vi "Read Dev Bounds.vi"(8 "error in (no error)":errorcluster, 11 "VISA resource name":refnum<visa-resource-name>) -> (0 "error out":errorcluster, 2 "dev bounds":T1, 3 "VISA resource name out":refnum<visa-resource-name>)   [LabVIEW 2019, in "Andeen-Hagerling 2700A.lvlib"]
doc: "Return the value of the deviation mode bounds parameters.\n\nThis is the upper and lower bounds of the deviation capacitance\nand loss spans in pF and jpF respectively. The capacitance\nand loss bounds correspond directly to the analog output\nvoltage bounds for capacitance and loss respectively."
uses:
  Andeen-Hagerling 2700A.lvlib
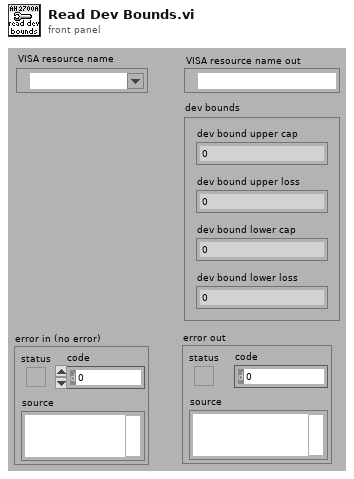
[diagram p1: front panel]
types:
  T1 = cluster{"dev bound upper cap":dbl, "dev bound upper loss":dbl, "dev bound lower cap":dbl, "dev bound lower loss":dbl}
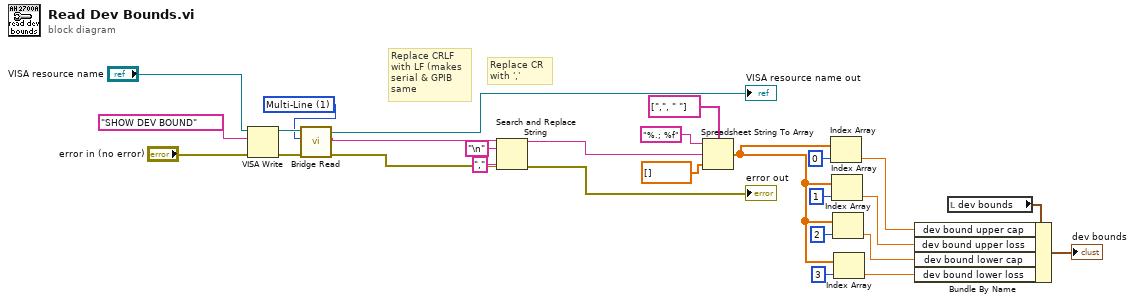
[diagram p0: block diagram]
diagram:
  w3 = u16 1 items=["Single Line", "Multi-Line"] ("Multiline")
  # "Replace CR\nwith ','"
  # "Replace CRLF\nwith LF (makes\nserial & GPIB \nsame"
  n1 = VISA Write(VISA resource name="VISA resource name", write buffer="SHOW DEV BOUND" ("command"), error in (no error)="error in (no error)") -> (VISA resource name out=w6:refnum<visa-resource-name>, error out=w5:errorcluster)  [unwired: 1 out]
  n2 = call "Bridge Read.vi"("error in (no error)"=w5, "multiline"=w3, "VISA resource name"=w6) -> ("error out"=w1:errorcluster, "read buffer"=w2:string, "VISA resource name out"=→"VISA resource name out":refnum<visa-resource-name>)  [unwired: 6 in]
  n3 = Search and Replace String(input string=w2, search string="\n", replace string="," ("replace string (\"\")"), error in=w1) -> (result string=w10:string, error out=→"error out":errorcluster)  [unwired: 4 in, 2 out]
  n4 = Spreadsheet String To Array(delimiter (Tab)=string[] [",", " "], format string="%.; %f", spreadsheet string=w10, array type (2D Dbl)=dbl[] []) -> (array=w18:dbl[])
  n5 = Index Array(array=w18, index=0) -> (element=w15:dbl)
  n6 = Index Array(array=w18, index=1) -> (element=w14:dbl)
  n7 = Index Array(array=w18, index=2) -> (element=w13:dbl)
  n8 = Index Array(array=w18, index=3) -> (element=w12:dbl)
  n9 = local read "dev bounds"() -> (w16:T1)
  n10 = Bundle By Name(cluster=w16, "dev bound upper cap"=w15, "dev bound upper loss"=w14, "dev bound lower cap"=w13, "dev bound lower loss"=w12) -> (→"dev bounds":T1)
